vi "Catch Process Error.vi"(8 "error in (no error)":errorcluster, 11 "priority action":string) -> (0 "error out":errorcluster, 3 "priority action":string)   [LabVIEW 2021, in "AudioGenUtility.lvlib"]
uses:
  AudioGenUtility.lvlib
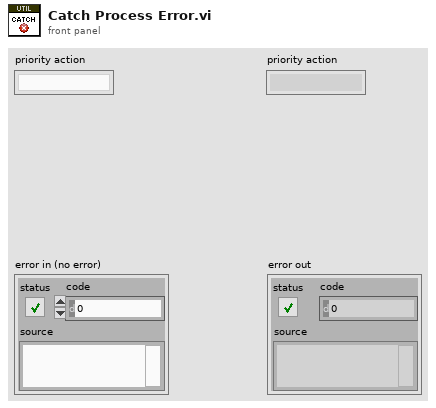
[diagram p1: front panel]
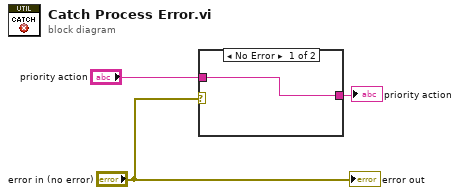
[diagram p0: block diagram]
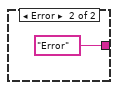
[diagram p2: hidden frame]
diagram:
  n1 = case shown="No Error" "error in (no error)" {
    tunnel: [w4 "Error"] -> w2
    tunnel: "priority action" -> [w4 _]
    frame No Error {
    }
    frame Error {
    }
  }
  "priority action" <- w2
  "error out" <- "error in (no error)"
